vi "Frame size U32 to frame size enum.vi"(1 "Frame Size U32":u32) -> (0 "Value":T1 items=["100X100"=100, "128X128"=128, "200X200"=200, "256X256"=256, "512X512"=512, "1024x1024"=1024, "2048x2048"=2048])   [LabVIEW 2013]
uses:
  Typedefs/Frame Size.ctl
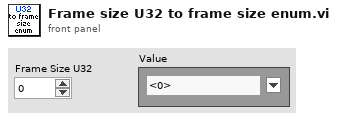
[diagram p1: front panel]
types:
  T1 = typedef "Frame Size.ctl" = u16
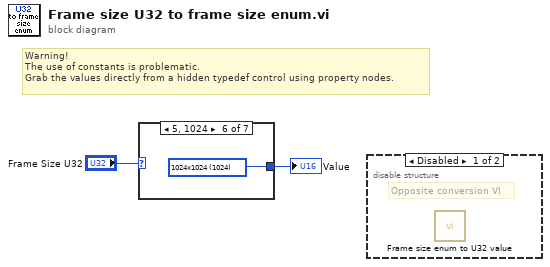
[diagram p0: block diagram]
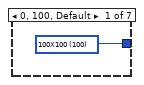
[diagram p3: hidden frame]
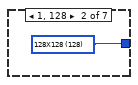
[diagram p4: hidden frame]
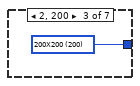
[diagram p5: hidden frame]
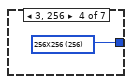
[diagram p6: hidden frame]
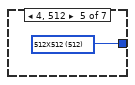
[diagram p7: hidden frame]
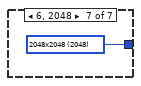
[diagram p8: hidden frame]
diagram:
  # "Warning!\nThe use of constants is problematic.\nGrab the values directly from a hidden typedef control using property nodes."
  n1 = case shown="5, 1024" "Frame Size U32" {
    tunnel: [w3 w4 w5 w6 w7 w8 w9] -> w1
    frame 0, 100, Default {
      w3 = T1 100 items=["100X100"=100, "128X128"=128, "200X200"=200, "256X256"=256, "512X512"=512, "1024x1024"=1024] ("Value 2")
    }
    frame 1, 128 {
      w4 = T1 128 items=["100X100"=100, "128X128"=128, "200X200"=200, "256X256"=256, "512X512"=512, "1024x1024"=1024] ("Value 2")
    }
    frame 2, 200 {
      w5 = T1 200 items=["100X100"=100, "128X128"=128, "200X200"=200, "256X256"=256, "512X512"=512, "1024x1024"=1024] ("Value 2")
    }
    frame 3, 256 {
      w6 = T1 256 items=["100X100"=100, "128X128"=128, "200X200"=200, "256X256"=256, "512X512"=512, "1024x1024"=1024] ("Value 2")
    }
    frame 4, 512 {
      w7 = T1 512 items=["100X100"=100, "128X128"=128, "200X200"=200, "256X256"=256, "512X512"=512, "1024x1024"=1024] ("Value 2")
    }
    frame 5, 1024 {
      w8 = T1 1024 items=["100X100"=100, "128X128"=128, "200X200"=200, "256X256"=256, "512X512"=512, "1024x1024"=1024] ("Value 2")
    }
    frame 6, 2048 {
      w9 = T1 2048 items=["100X100"=100, "128X128"=128, "200X200"=200, "256X256"=256, "512X512"=512, "1024x1024"=1024, "2048x2048"=2048] ("Value 2")
    }
  }
  "Value" <- w1
  n2 = disable-structure shown="Disabled" {
    frame Disabled {
      # "Opposite conversion VI"
      n3 = call "Frame size enum to U32 value.vi"() -> ()  [unwired: 1 in, 1 out]
    }
    frame Enabled {
    }
  }
